vi "Inject OAuth Client Type.vi"(10 "OAuthClient":refnum<class "OAuthClient.lvclass">, 11 "Oauth2 in":refnum<class "Oauth2.lvclass">) -> (3 "Oauth2":refnum<class "Oauth2.lvclass">)   [LabVIEW 2020, in "Oauth2.lvclass"]
uses:
  Oauth2.lvclass
  OauthClient/OAuthClient.lvclass
  Oauth2.lvclass/Oauth2.ctl
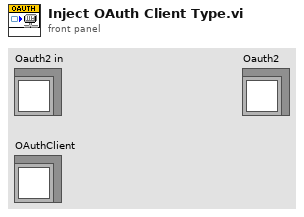
[diagram p1: front panel]
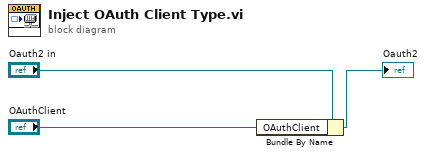
[diagram p0: block diagram]
diagram:
  n1 = Bundle By Name(cluster="Oauth2 in", "OAuthClient"="OAuthClient") -> (→"Oauth2":refnum<class "Oauth2.lvclass">)
